vi "Data_get.vi"() -> ()   [LabVIEW 2009]
uses:
  <vilib>/Analysis/2dsp.llb/Real FFT.vi
  <vilib>/Analysis/NI_AALPro.lvlib
panel:
  in  "Substr":bool
  out "tdsavges#":i32 caption="tds averaged:"
  in  "Auto":bool caption="Autosave"
  in  "FFT every#":u32=1 min=1 max=1000 step=1
  in  "#steps":u32=1 min=1 step=1
  in  "f step (MHz)":dbl=0.0003 min=0.00025 max=67.0 step=1e-06 format="%#.12f"
  in  "ps/point":T1(ring)
  in  "ns/div":T2(ring)
  out "Current sweep":u32=1 min=1 max=1000 step=1
  in  "Ext":string="ccd"
  out "f cur. (MHz)":string
  in  "Name":string="trace"
  in  "Folder":path
  in  "#Sweeps":u32=1 min=1 max=1000 step=1
  in  "Ampl. (dBm)":dbl min=-135.0 max=30.0 step=0.5 format="%#_8g"
  in  "f start (MHz)":dbl=0.0003 min=0.00025 max=67.0 step=1e-06 format="%#.12f"
  in  "Start":bool
  in  "Quit":bool
  in  "E8257D VISA Port":refnum<visa-resource-name>="GPIB0::1::INSTR"
  out "read time (ms)":u32
  out "#points":u32
  out "Busy":bool
  in  "Repetition rate (Hz)":ext=2.5
  in  "Chirp start (MHz)":ext=2.5
  in  "Filter up to (MHz)":ext=2.5
  in  "Amount of averagings":u32=10
  out "Data":dbl[](array[numeric])
  out "XY Graph 5":cluster{ext[], dbl[]}(graph)
  out "FFT (Im)":dbl[](array[numeric])
  out "FFT (Re)":dbl[](array[numeric])
  out "Final array":ext[][](array[numeric])
  out "size(s)":i32
  out "Oscilloscope Data":dbl[](array[numeric])
  in  "Channel Number":u16=1
  out "Oscilloscope graph":dbl[](graph)
  in  "Stop":bool
  in  "TDS VISA Port":refnum<visa-resource-name>="GPIB0::1::INSTR"
  # "TDS6000"
  # "E8257D"
  # "File Storage"
  # "Control"
  # "Spectrum data"
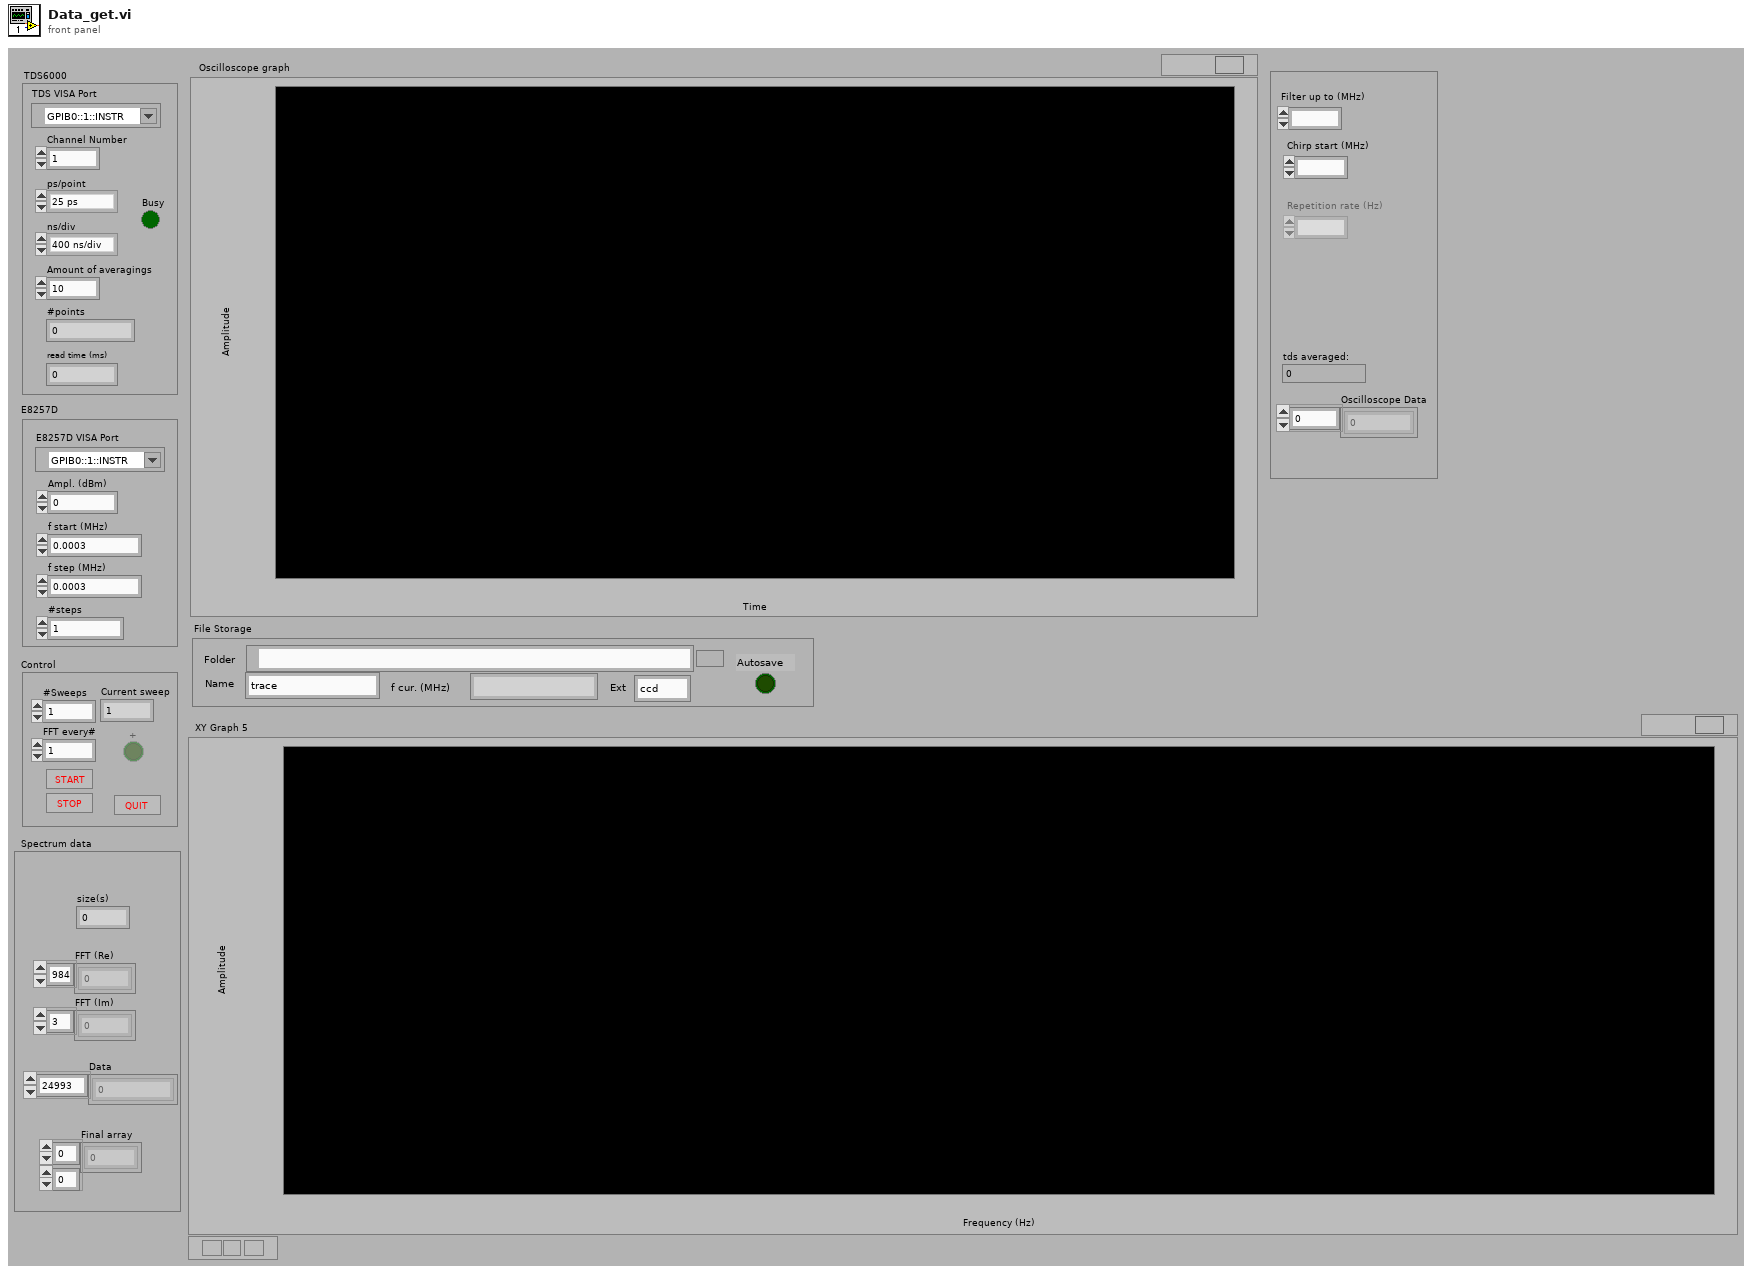
[diagram p1: front panel]
types:
  T1 = enum16{"25 ps", "50 ps", "100 ps", "200 ps", "400 ps", "800 ps", "2 ns"}
  T2 = enum16{"400 ns/div", "1 us/div", "2 us/div", "4 us/div", "10 us/div", "20 us/div"}
  T3 = enum16{"open", "replace", "create", "open or create", "replace or create", "replace or create with confirmation"}
  T4 = cluster{"Folder":path, "Name":string, "Ext":string}
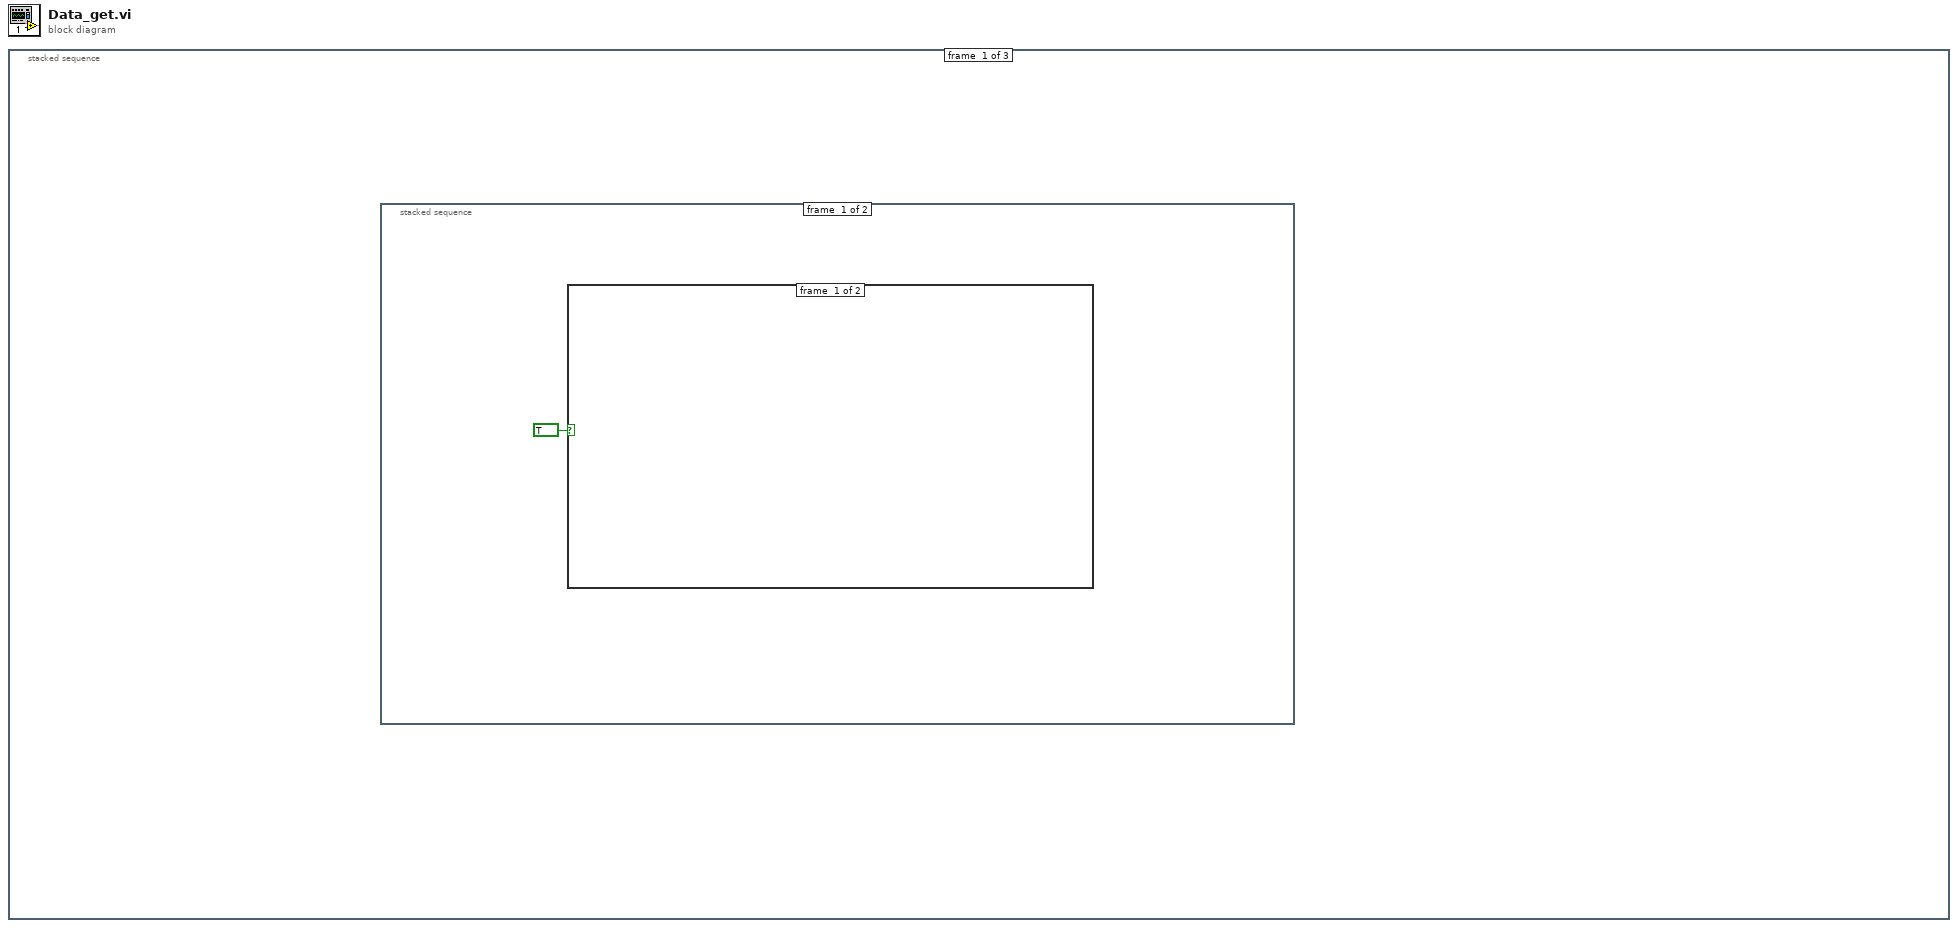
[diagram p0: block diagram]
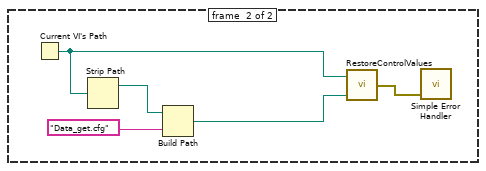
[diagram p2: hidden frame]
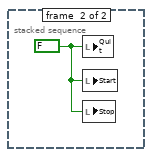
[diagram p3: hidden frame]
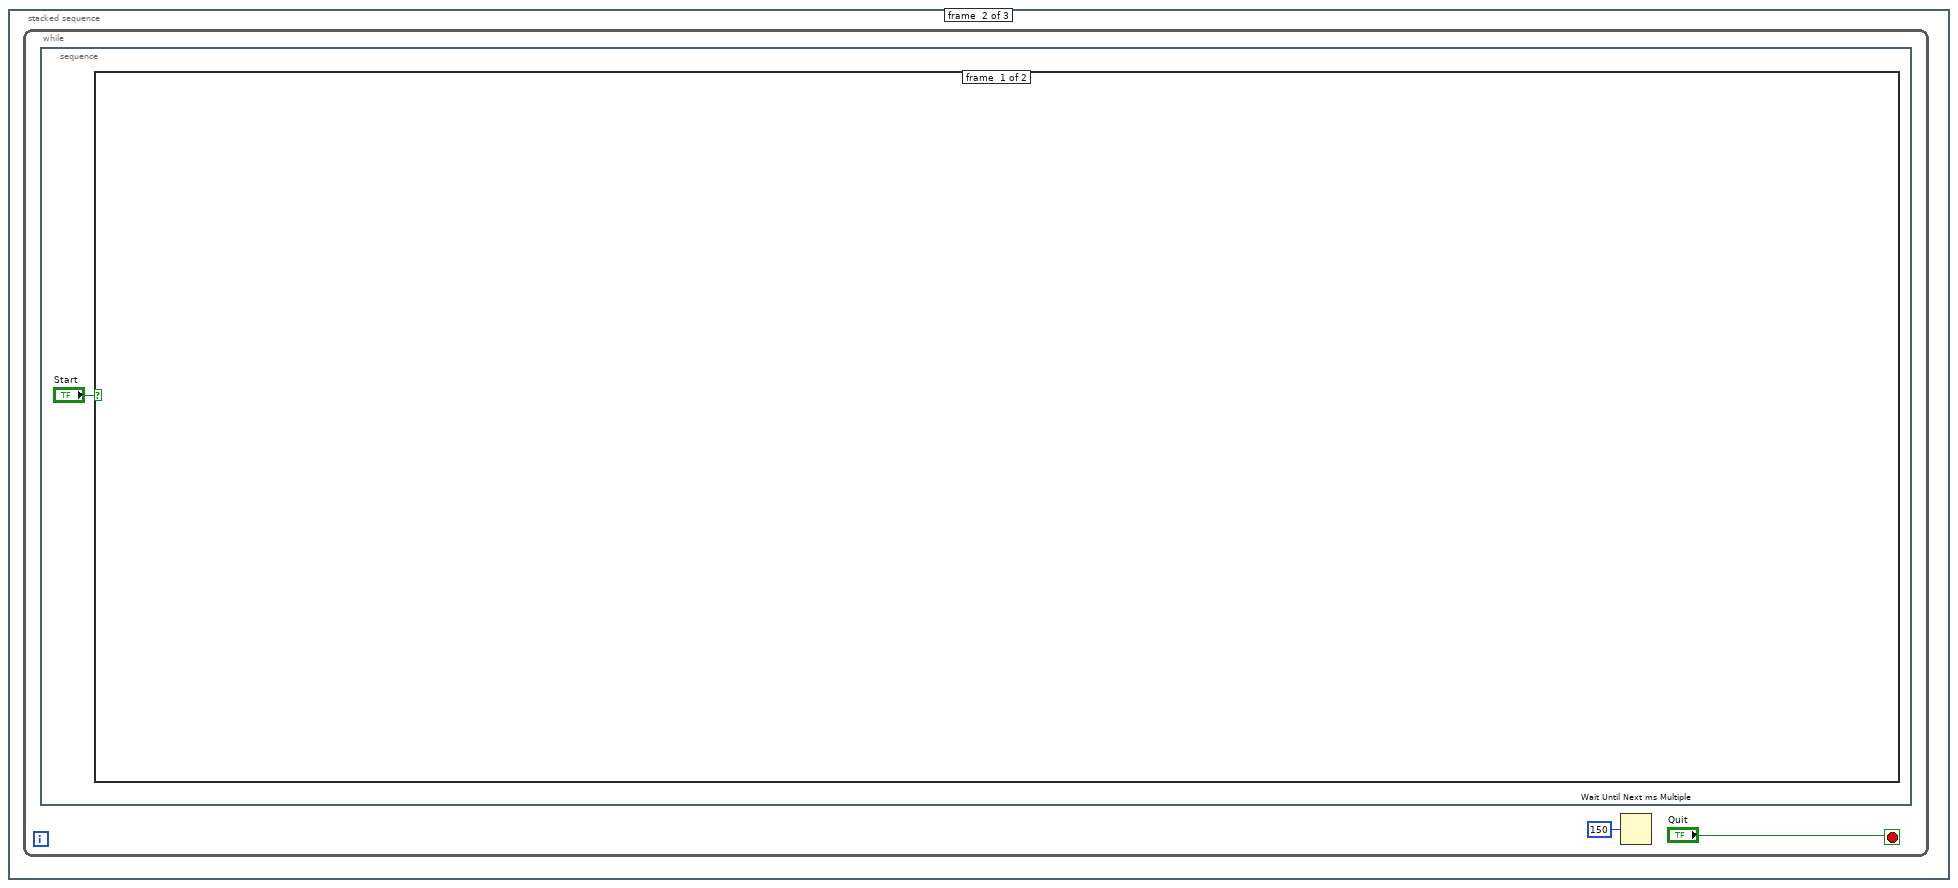
[diagram p4: hidden frame]
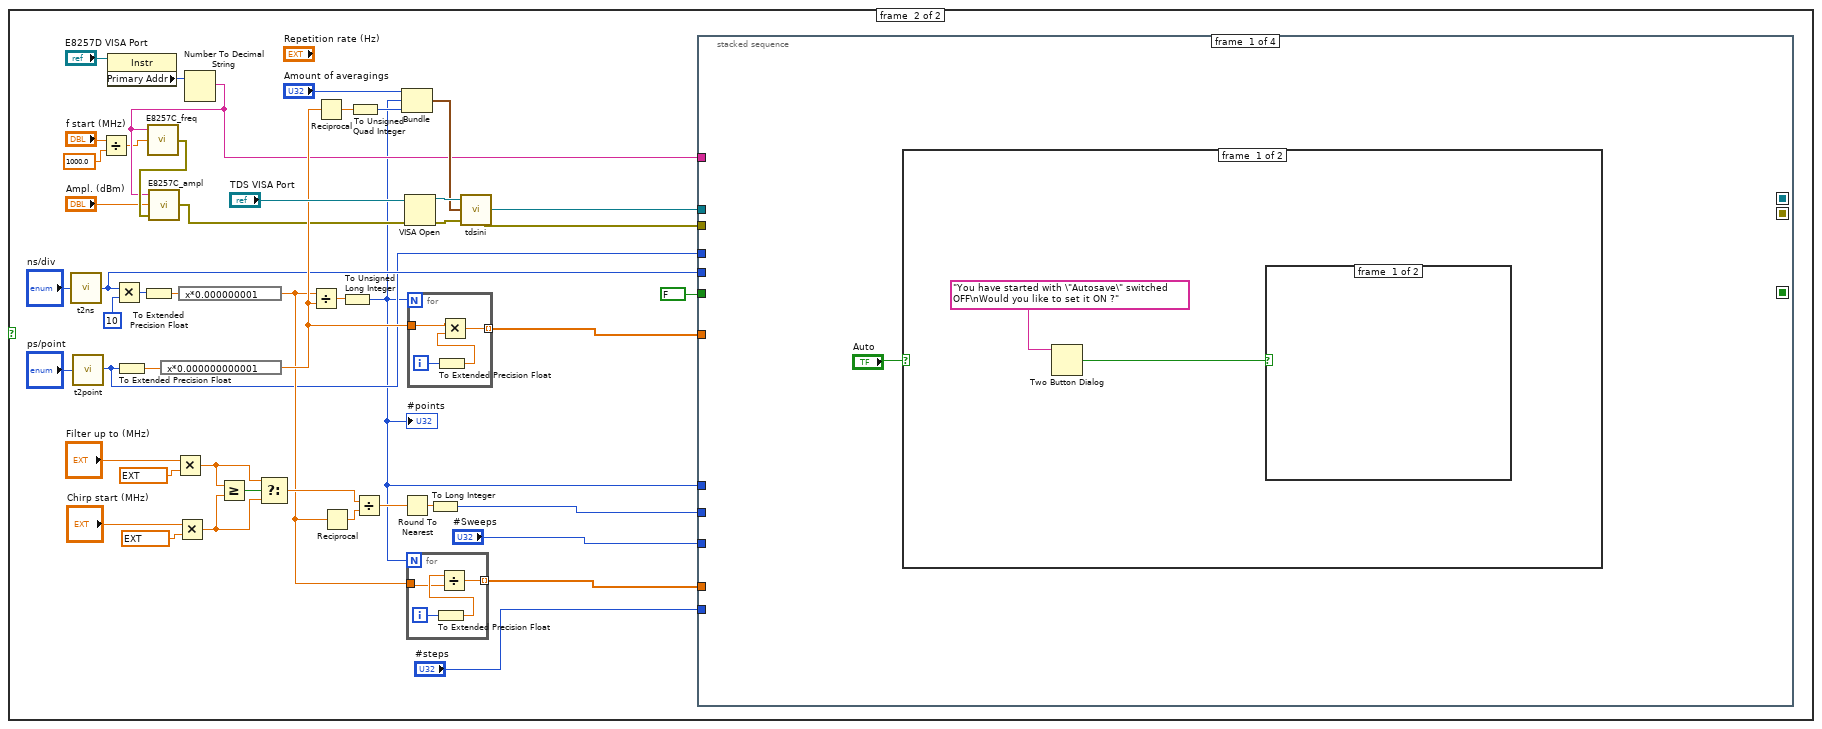
[diagram p5: hidden frame]
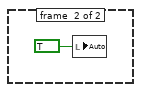
[diagram p6: hidden frame]
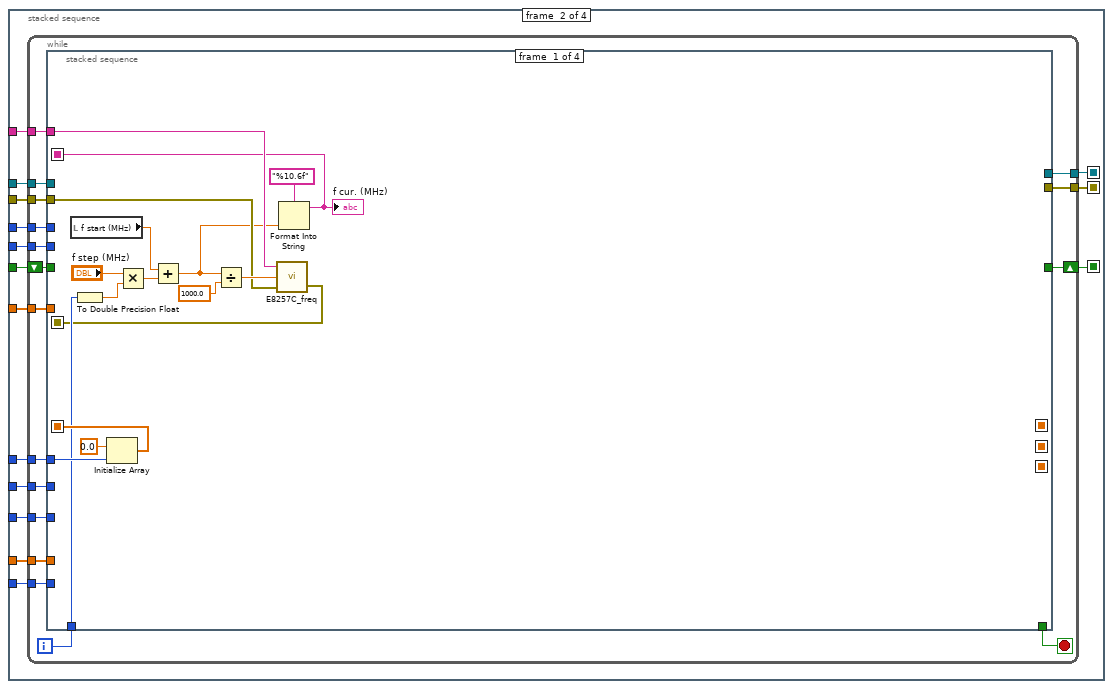
[diagram p8: hidden frame]
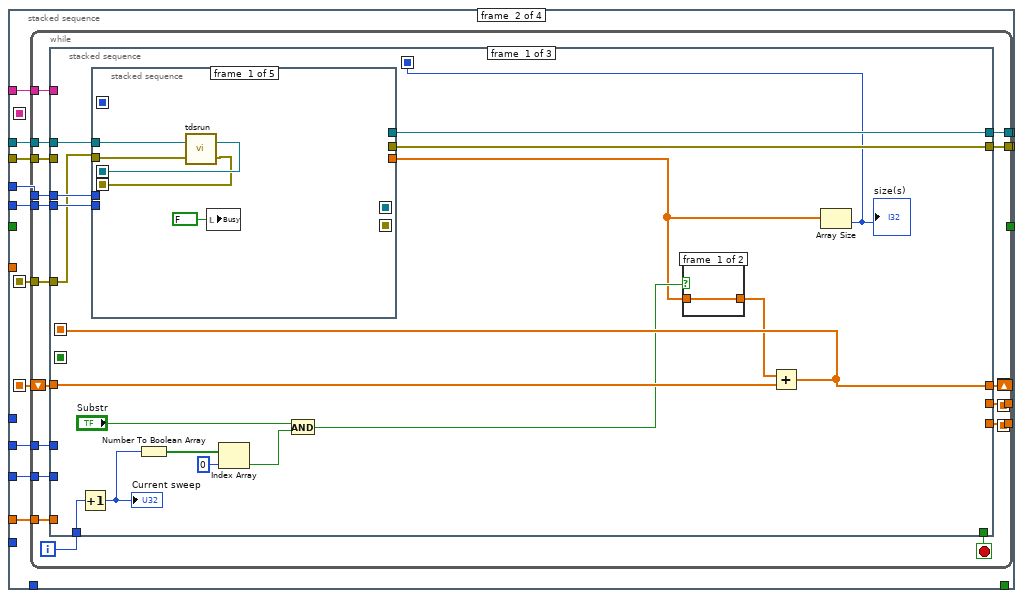
[diagram p9: hidden frame]
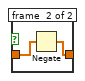
[diagram p10: hidden frame]
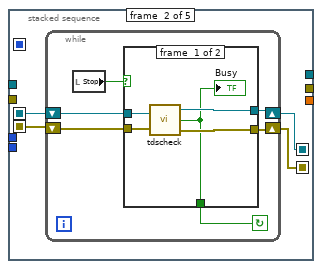
[diagram p11: hidden frame]
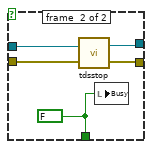
[diagram p12: hidden frame]
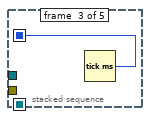
[diagram p13: hidden frame]
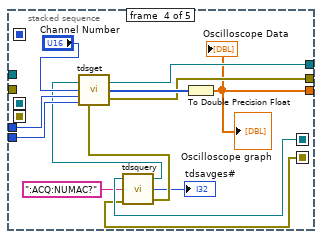
[diagram p14: hidden frame]
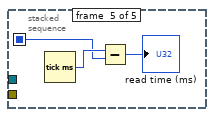
[diagram p15: hidden frame]
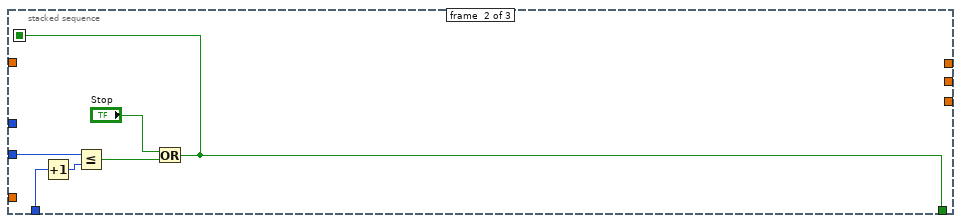
[diagram p16: hidden frame]
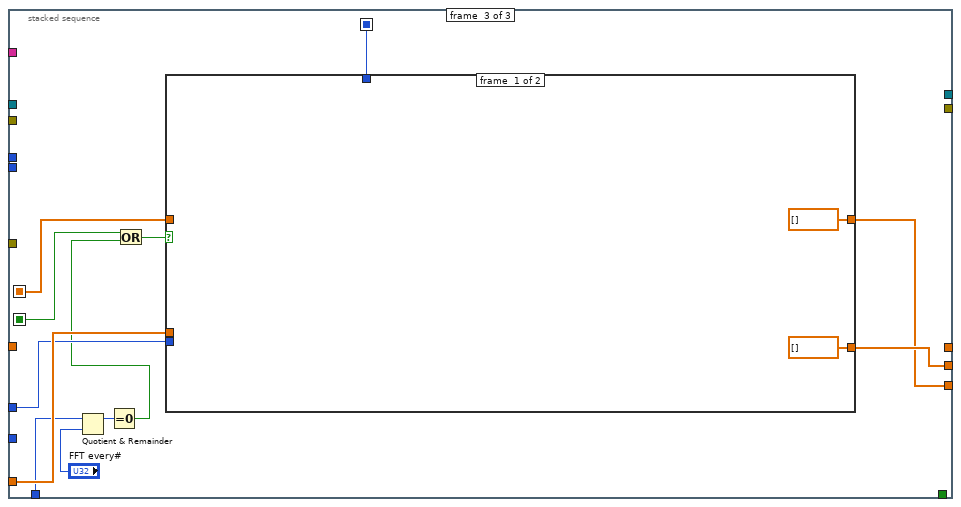
[diagram p17: hidden frame]
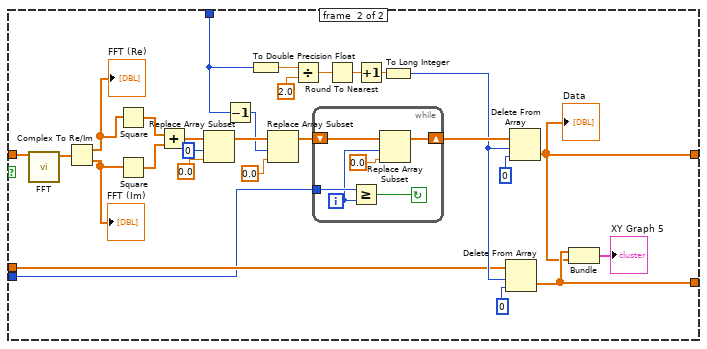
[diagram p18: hidden frame]
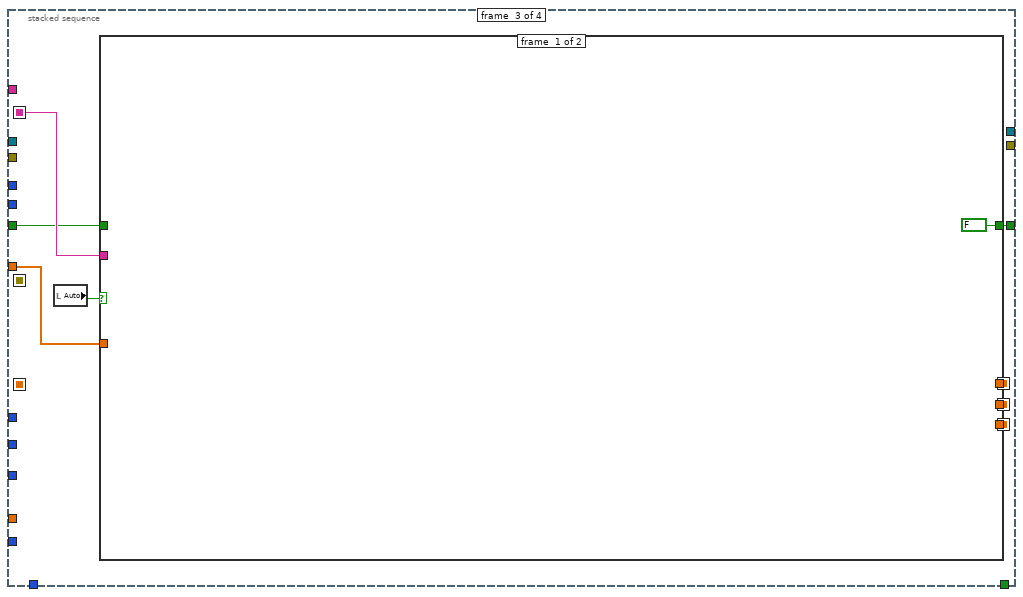
[diagram p19: hidden frame]
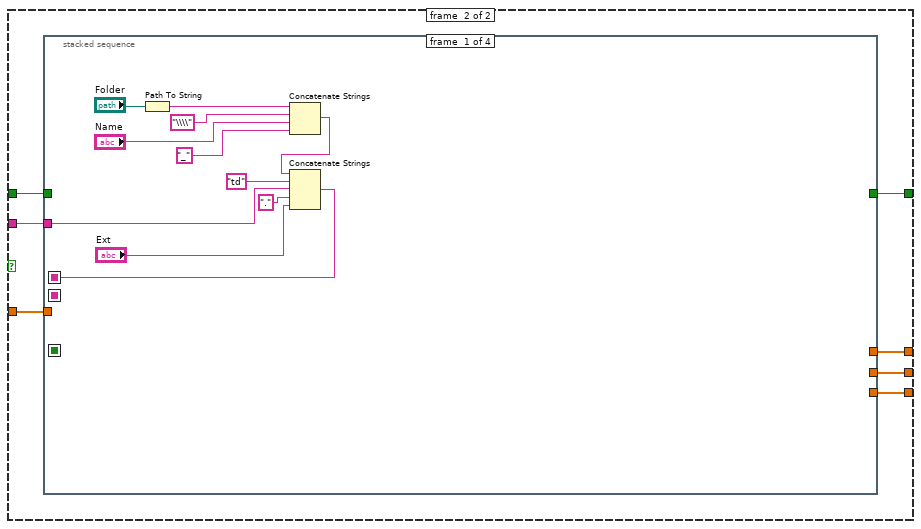
[diagram p20: hidden frame]
diagram:
  n1 = stacked-sequence {
    frame #0 {
      n2 = stacked-sequence {
        frame #0 {
          n3 = case shown="True" TRUE {
            frame #0 {
            }
            frame #1 {
              n4 = Current VI's Path() -> (path=w2:path)
              n5 = Strip Path(path=w2) -> (stripped path=w3:path)  [unwired: 1 out]
              n6 = Build Path(base path=w3, name or relative path="Data_get.cfg") -> (appended path=w5:path)
              n7 = call "RestoreControlValues.vi"("file path"=w5, "vi path"=w2) -> ("error out"=w4:errorcluster)
              n8 = call <vilib>:"Simple Error Handler.vi"("error in (no error)"=w4) -> ()  [unwired: 4 in, 5 out]
            }
          }
        }
        frame #1 {
          w7 = FALSE ("Quit")
          n9 = local write "Quit"(w7) -> ()
          n10 = local write "Start"(w7) -> ()
          n11 = local write "Stop"(w7) -> ()
        }
      }
    }
    frame #1 {
      n12 = while {
        stop <- "Quit" stop-if-true
        n13 = stacked-sequence {
          frame #0 {
            n14 = case shown="True" "Start" {
              frame #0 {
              }
              frame #1 {
                n15 = call "t2ns.vi"("t/div"="ns/div") -> ("ns/div"=w17:u32)
                n16 = call "t2point.vi"("t/point"="ps/point") -> ("ps/point"=w15:u32)
                n17 = Divide(x="f start (MHz)", y=1000.0) -> (x/y=w20:dbl)
                n18 = property class="Instr"(reference="E8257D VISA Port") -> ("Primary Addr"=w27:u16)  [unwired: 1 in, 2 out]
                n19 = Multiply(x=w17, y=u32 10) -> (x*y=w51:u32)
                n20 = To Extended Precision Float(1:w15) -> (0:w48:ext)
                n21 = To Extended Precision Float(1:w51) -> (0:w49:ext)
                n22 = expression code="x*0.000000000001"(w48) -> (w33:ext)
                n23 = Multiply(x="Filter up to (MHz)", y=ext 1000000.0) -> (x*y=w39:ext)
                n24 = Multiply(x="Chirp start (MHz)", y=ext 1000000.0) -> (x*y=w36:ext)
                n25 = expression code="x*0.000000001"(w49) -> (w29:ext)
                n26 = Number To Decimal String(number=w27) -> (decimal integer string=w24:string)  [unwired: 1 in]
                n27 = call "E8257C_freq.vi"("Frequency GHz"=w20, "GPIB address"=w24) -> ("error out"=w25:errorcluster)  [unwired: 1 in]
                n28 = call "E8257C_ampl.vi"("error in"=w25, "Amplitude dBm"="Ampl. (dBm)", "GPIB address"=w24) -> ("error out"=w23:errorcluster)
                n29 = Greater Or Equal?(x=w39, y=w36) -> (x >= y?=w47:bool)
                n30 = Select(t=w39, s=w47, f=w36) -> (s? t:f=w45:ext)
                n31 = Divide(x=w29, y=w33) -> (x/y=w50:ext)
                n32 = Reciprocal(x=w33) -> (1/x=w31:ext)
                n33 = Reciprocal(x=w29) -> (1/x=w46:ext)
                n34 = To Unsigned Long Integer(number=w50) -> (unsigned 32bit integer=w13:u32)
                "#points" <- w13
                n35 = To Unsigned Quad Integer(1:w31) -> (0:w32:u64)
                n36 = Divide(x=w45, y=w46) -> (x/y=w44:ext)
                n37 = Bundle("Amount of averagings"="Amount of averagings", w13, w32) -> (w34:cluster{"Amount of averagings ":u32, u32, u64})  [unwired: 1 in]
                n38 = Round To Nearest(number=w44) -> (nearest integer value=w43:ext)
                n39 = VISA Open(error in (no error)=w23, VISA resource name="TDS VISA Port") -> (VISA resource name=w54:refnum<visa-resource-name>, error out=w55:errorcluster)  [unwired: 3 in]
                n40 = for {
                  N: w13 -> [_]
                  tunnel: w29 -> [w433]
                  tunnel: [w435] -> w30 mode=indexing
                  i -> [w436]
                  n41 = To Extended Precision Float(1:w436) -> (0:w434:ext)
                  n42 = Divide(x=w434, y=w433) -> (x/y=w435:ext)
                }
                n43 = for {
                  N: w13 -> [_]
                  tunnel: w33 -> [w438]
                  tunnel: [w437] -> w18 mode=indexing
                  i -> [w440]
                  n44 = To Extended Precision Float(1:w440) -> (0:w439:ext)
                  n45 = Multiply(x=w438, y=w439) -> (x*y=w437:ext)
                }
                n46 = To Long Integer(number=w43) -> (32bit integer=w42:i32)
                n47 = call "tdsini.vi"("Error In (No Error)"=w55, "Acq_par"=w34, "VISA Port In"=w54) -> ("Error Out"=w56:errorcluster, "VISA Port Out"=w57:refnum<visa-resource-name>)
                n48 = stacked-sequence {
                  seq-local: [_ w68 _ _] -> [_ _ w394 _]
                  seq-local: [_ w67 _ _] -> [_ _ w393 _]
                  seq-local: [_ w62 _ _] -> [_ _ _ w395]
                  tunnel: w57 -> [_ w76 _ _]
                  tunnel: w56 -> [_ w75 _ _]
                  tunnel: w15 -> [_ w74 _ _]
                  tunnel: w17 -> [_ w73 _ _]
                  tunnel: w42 -> [_ w72 _ _]
                  tunnel: w30 -> [_ w71 _ _]
                  tunnel: w24 -> [_ w70 w391 _]
                  tunnel: "#Sweeps" -> [_ w69 _ _]
                  tunnel: w18 -> [_ w64 _ _]
                  tunnel: w13 -> [_ w66 _ _]
                  tunnel: "#steps" -> [_ w65 _ _]
                  tunnel: FALSE -> [_ w63 _ _]
                  frame #0 {
                    n49 = case shown="False" "Auto" {
                      frame #0 {
                        n50 = Two Button Dialog(message="You have started with \"Autosave\" switched OFF\nWould you like to set it ON ?") -> (T button?=w59:bool)  [unwired: 2 in]
                        n51 = case shown="True" w59 {
                          frame #0 {
                          }
                          frame #1 {
                            n52 = local write "Auto"(TRUE) -> ()
                          }
                        }
                      }
                      frame #1 {
                      }
                    }
                  }
                  frame #1 {
                    n53 = while {
                      tunnel: w76 -> [w93]
                      tunnel: w75 -> [w92]
                      tunnel: w74 -> [w91]
                      tunnel: w73 -> [w90]
                      tunnel: w72 -> [w89]
                      tunnel: w71 -> [w88]
                      tunnel: w70 -> [w87]
                      tunnel: w69 -> [w86]
                      tunnel: [w85] -> w68
                      tunnel: [w84] -> w67
                      tunnel: w66 -> [w83]
                      tunnel: w65 -> [w81]
                      tunnel: w64 -> [w79]
                      shift-right: [w77] -> w62
                      shift-left: w63 -> [w78]
                      i -> [w82]
                      stop <- w80 stop-if-true
                      n54 = stacked-sequence {
                        seq-local: [w108 _ _ _] -> [_ w114 _ _]
                        seq-local: [w97 _ _ _] -> [_ w113 _ _]
                        seq-local: [_ w112 _ _] -> [_ _ w265 _]
                        seq-local: [_ w111 _ _] -> [_ _ w264 _]
                        seq-local: [_ w110 _ _] -> [_ _ w263 _]
                        seq-local: [w94 _ _ _] -> [_ _ w262 _]
                        tunnel: w93 -> [_ w124 _ _]
                        tunnel: w92 -> [w98 w123 _ _]
                        tunnel: w91 -> [_ w122 _ _]
                        tunnel: w90 -> [_ w121 _ _]
                        tunnel: w89 -> [_ w120 _ _]
                        tunnel: w88 -> [_ w119 _ _]
                        tunnel: w87 -> [w99 w118 _ _]
                        tunnel: w86 -> [_ w117 _ _]
                        tunnel: [_ w116 _ _] -> w85
                        tunnel: [_ w115 _ _] -> w84
                        tunnel: w83 -> [w107 _ _ _]
                        tunnel: w82 -> [w102 _ _ w387]
                        tunnel: w81 -> [_ _ _ w386]
                        tunnel: [_ _ _ w385] -> w80
                        tunnel: w79 -> [_ _ w266 _]
                        tunnel: w78 -> [_ _ w260 _]
                        tunnel: [_ _ w259 _] -> w77
                        frame #0 {
                          n55 = local read "f start (MHz)"() -> (w100:dbl)
                          n56 = To Double Precision Float(number=w102) -> (double precision float=w103:dbl)
                          n57 = Initialize Array(0.0 ("element"), w107) -> (w108:dbl[])
                          n58 = Multiply(x="f step (MHz)", y=w103) -> (x*y=w101:dbl)
                          n59 = Add(x=w100, y=w101) -> (x+y=w96:dbl)
                          n60 = Divide(x=w96, y=1000.0) -> (x/y=w106:dbl)
                          n61 = call "E8257C_freq.vi"("error in"=w98, "Frequency GHz"=w106, "GPIB address"=w99) -> ("error out"=w97:errorcluster)
                          n62 = Format Into String(format string="%10.6f", w96) -> (resulting string=w94:string)  [unwired: 2 in, 1 out]
                          "f cur. (MHz)" <- w94
                        }
                        frame #1 {
                          n63 = while {
                            tunnel: [w138] -> w115
                            tunnel: [w139] -> w116
                            tunnel: w123 -> [w140]
                            tunnel: w124 -> [w141]
                            tunnel: w122 -> [w137]
                            tunnel: w121 -> [w136]
                            tunnel: w119 -> [w134]
                            tunnel: w120 -> [w135]
                            tunnel: w118 -> [w131]
                            tunnel: w117 -> [w130]
                            shift-right: [w128] -> w112
                            shift-left: w114 -> [w129]
                            tunnel: [w127] -> w111
                            tunnel: w113 -> [w126]
                            tunnel: [w125] -> w110
                            i -> [w133]
                            stop <- w132 stop-if-true
                            n64 = stacked-sequence {
                              seq-local: [w151 _ _] -> [_ _ w222]
                              seq-local: [w152 _ _] -> [_ _ w221]
                              seq-local: [_ w205 _] -> [_ _ w212]
                              tunnel: w141 -> [w159 _ _]
                              tunnel: w140 -> [_ _ _]
                              tunnel: [w158 _ _] -> w139
                              tunnel: [w157 _ _] -> w138
                              tunnel: w137 -> [w156 _ _]
                              tunnel: w136 -> [w155 _ _]
                              tunnel: w135 -> [_ _ w219]
                              tunnel: w134 -> [_ _ w220]
                              tunnel: w133 -> [w150 w210 w216]
                              tunnel: [_ w205 _] -> w132
                              tunnel: w131 -> [_ _ _]
                              tunnel: w130 -> [_ w207 _]
                              tunnel: w129 -> [w154 _ _]
                              tunnel: [w152 _ _] -> w128
                              tunnel: [_ _ w218] -> w127
                              tunnel: w126 -> [w153 _ _]
                              tunnel: [_ _ w217] -> w125
                              frame #0 {
                                n65 = Increment(x=w150) -> (x+1=w142:i32)
                                "Current sweep" <- w142
                                n66 = stacked-sequence {
                                seq-local: [w165 _ _ _ _] -> [_ w171 _ _ _]
                                seq-local: [w164 _ _ _ _] -> [_ w170 _ _ _]
                                seq-local: [_ w168 _ _ _] -> [_ _ _ w193 _]
                                seq-local: [_ w169 _ _ _] -> [_ _ _ w194 _]
                                seq-local: [_ _ w188 _ _] -> [_ _ _ _ w203]
                                tunnel: w159 -> [w166 _ _ _ _]
                                tunnel: w153 -> [w167 _ _ _ _]
                                tunnel: [_ _ _ w200 _] -> w158
                                tunnel: [_ _ _ w199 _] -> w157
                                tunnel: w156 -> [_ _ _ w197 _]
                                tunnel: w155 -> [_ _ _ w196 _]
                                tunnel: [_ _ _ w195 _] -> w145
                                frame #0 {
                                n67 = call "tdsrun.vi"("Error In (No Error)"=w167, "VISA Port In"=w166) -> ("Error Out"=w164:errorcluster, "VISA Port Out"=w165:refnum<visa-resource-name>)
                                n68 = local write "Busy"(FALSE ("Busy")) -> ()
                                }
                                frame #1 {
                                n69 = while {
                                shift-right: [w175] -> w169
                                shift-left: w171 -> [w176]
                                shift-right: [w174] -> w168
                                shift-left: w170 -> [w177]
                                stop <- w173 continue-if-true
                                n70 = local read "Stop"() -> (w172:bool)
                                n71 = case shown="True" w172 {
                                tunnel: w177 -> [w182 w186]
                                tunnel: w176 -> [w181 w187]
                                tunnel: [w180 w184] -> w175
                                tunnel: [w179 w185] -> w174
                                tunnel: [w178 w183] -> w173
                                frame #0 {
                                n72 = call "tdscheck.vi"("VISA Port In"=w181, "Error In (No Error)"=w182) -> ("VISA Port Out"=w180:refnum<visa-resource-name>, "busy"=w178:bool, "Error Out"=w179:errorcluster)
                                "Busy" <- w178
                                }
                                frame #1 {
                                w183 = FALSE ("busy")
                                n73 = call "tdsstop.vi"("Error In (No Error)"=w186, "VISA Port In"=w187) -> ("Error Out"=w185:errorcluster, "VISA Port Out"=w184:refnum<visa-resource-name>)
                                n74 = local write "Busy"(w183) -> ()
                                }
                                }
                                }
                                }
                                frame #2 {
                                n75 = Tick Count (ms)() -> (millisecond timer value=w188:u32)
                                }
                                frame #3 {
                                n76 = call "tdsquery.vi"("Error In (No Error)"=w193, "String to TDS"=":ACQ:NUMAC?", "VISA Port In"=w194) -> ("Error Out"=w190:errorcluster, "number"=→"tdsavges#":i32, "VISA Port Out"=w191:refnum<visa-resource-name>)
                                n77 = call "tdsget.vi"("VISA Port In"=w191, "Channel Number"="Channel Number", "ps/point"=w197, "ns/div"=w196, "Error In (No Error)"=w190) -> ("VISA Port Out"=w200:refnum<visa-resource-name>, "TDS Data"=w201:u16[], "Error Out"=w199:errorcluster)  [unwired: 8 in]
                                n78 = To Double Precision Float(number=w201) -> (double precision float=w195:dbl[])
                                "Oscilloscope graph" <- w195
                                "Oscilloscope Data" <- w195
                                }
                                frame #4 {
                                n79 = Tick Count (ms)() -> (millisecond timer value=w204:u32)
                                n80 = Subtract(x=w204, y=w203) -> (x-y=→"read time (ms)":u32)
                                }
                                }
                                n81 = Number To Boolean Array(number=w142) -> (Boolean array=w149:bool[])
                                n82 = Index Array(array=w149, index=0) -> (element=w147:bool)
                                n83 = And(x="Substr", y=w147) -> (x .and. y?=w146:bool)
                                n84 = case shown="True" w146 {
                                tunnel: w145 -> [w160 w162]
                                tunnel: [w160 w161] -> w144
                                frame #0 {
                                }
                                frame #1 {
                                n85 = Negate(x=w162) -> (-x=w161:dbl[])
                                }
                                }
                                n86 = Add(x=w144, y=w154) -> (x+y=w152:dbl[])
                                n87 = Array Size(array=w145) -> (size(s)=w151:i32)
                                "size(s)" <- w151
                              }
                              frame #1 {
                                n88 = Increment(x=w210) -> (x+1=w206:i32)
                                n89 = Less Or Equal?(x=w207, y=w206) -> (x <= y?=w209:bool)
                                n90 = Or(x="Stop", y=w209) -> (x .or. y?=w205:bool)
                              }
                              frame #2 {
                                n91 = Quotient & Remainder(x=w216, y="FFT every#") -> (x-y*floor(x/y)=w214:u32)  [unwired: 1 out]
                                n92 = Equal To 0?(x=w214) -> (x = 0?=w211:bool)
                                n93 = Or(x=w212, y=w211) -> (x .or. y?=w213:bool)
                                n94 = case shown="True" w213 {
                                tunnel: w222 -> [_ w230]
                                tunnel: w221 -> [_ w229]
                                tunnel: w220 -> [_ w228]
                                tunnel: w219 -> [_ w227]
                                tunnel: [ext[] [] w226] -> w218
                                tunnel: [dbl[] [] w225] -> w217
                                frame #0 {
                                }
                                frame #1 {
                                n95 = call-poly <vilib>:"FFT.vi"("X"=w229) -> ("FFT {X}"=w252:cdb[])  [unwired: 9 in, 1 out]
                                n96 = Complex To Re/Im(x + iy=w252) -> (x=w251:dbl[], y=w250:dbl[])
                                "FFT (Re)" <- w251
                                "FFT (Im)" <- w250
                                n97 = Square(x=w251) -> (x^2=w249:dbl[])
                                n98 = Square(x=w250) -> (x^2=w248:dbl[])
                                n99 = Add(x=w249, y=w248) -> (x+y=w244:dbl[])
                                n100 = Replace Array Subset(array=w244, new element=0.0 ("new element/subarray"), index=0) -> (w243:dbl[])
                                n101 = Decrement(x=w230) -> (x-1=w242:i32)
                                n102 = To Double Precision Float(number=w230) -> (double precision float=w238:dbl)
                                n103 = Replace Array Subset(array=w243, new element=0.0 ("new element/subarray"), index=w242) -> (w240:dbl[])
                                n104 = Divide(x=w238, y=2.0) -> (x/y=w236:dbl)
                                n105 = while {
                                tunnel: w227 -> [w257]
                                shift-right: [w255] -> w239
                                shift-left: w240 -> [w256]
                                i -> [w254]
                                stop <- w258 continue-if-true
                                n106 = Greater Or Equal?(x=w257, y=w254) -> (x >= y?=w258:bool)
                                n107 = Replace Array Subset(array=w256, new element=0.0 ("new element/subarray"), index=w254) -> (w255:dbl[])
                                }
                                n108 = Round To Nearest(number=w236) -> (nearest integer value=w235:dbl)
                                n109 = Increment(x=w235) -> (x+1=w234:dbl)
                                n110 = To Long Integer(number=w234) -> (32bit integer=w231:i32)
                                n111 = Delete From Array(array=w228, length=w231, index=0) -> (deleted portion=w226:ext[])  [unwired: 1 out]
                                n112 = Delete From Array(array=w239, length=w231, index=0) -> (deleted portion=w225:dbl[])  [unwired: 1 out]
                                "Data" <- w225
                                n113 = Bundle(w226, w225) -> (→"XY Graph 5":cluster{ext[], dbl[]})  [unwired: 1 in]
                                }
                                }
                              }
                            }
                          }
                        }
                        frame #2 {
                          n114 = local read "Auto"() -> (w261:bool)
                          n115 = case shown="True" w261 {
                            tunnel: w266 -> [_ w274]
                            tunnel: w265 -> [_ w273]
                            tunnel: w264 -> [_ w272]
                            tunnel: w263 -> [_ w271]
                            tunnel: w262 -> [_ w270]
                            tunnel: w260 -> [_ w269]
                            tunnel: [FALSE w268] -> w259
                            frame #0 {
                            }
                            frame #1 {
                              n116 = stacked-sequence {
                                seq-local: [w275 _ _ _] -> [_ w300 _ _]
                                seq-local: [_ _ w355 _] -> [_ _ _ w376]
                                seq-local: [_ w287 _ _] -> [_ _ _ w367]
                                tunnel: w274 -> [_ w302 _ _]
                                tunnel: w273 -> [_ w289 _ _]
                                tunnel: w272 -> [_ _ _ w379]
                                tunnel: w271 -> [_ _ _ w378]
                                tunnel: w270 -> [w277 w288 w357 _]
                                tunnel: w269 -> [_ w292 _ _]
                                tunnel: [_ w287 _ _] -> w268
                                frame #0 {
                                n117 = Path To String(path="Folder") -> (string=w285:string)
                                n118 = Concatenate Strings(w285, "\\\\" ("string"), "Name", "_") -> (w276:string)
                                n119 = Concatenate Strings(w276, "td", w277, ".", "Ext") -> (w275:string)
                                }
                                frame #1 {
                                n120 = String To Path(string=w300) -> (path=w291:path)
                                n121 = case shown="False" w292 {
                                tunnel: w300 -> [w306 _]
                                tunnel: [w311 w353] -> w287
                                tunnel: [w309 T3."replace or create" ("operation (0:open)")] -> w294
                                tunnel: w292 -> [w310 w353]
                                tunnel: w291 -> [w308 w352]
                                tunnel: [w307 w352] -> w290
                                tunnel: w288 -> [w305 _]
                                frame #0 {
                                n122 = call "CheckFileExist.vi"("Path"=w306) -> ("Exist"=w313:bool, "Overwrite"=w312:bool)  [unwired: 1 in, 1 out]
                                n123 = case shown="True" w313 {
                                tunnel: w312 -> [_ w322]
                                tunnel: [w316 w320] -> w311
                                tunnel: w310 -> [w316 _]
                                tunnel: [T3."create" ("operation (0:open)") w321] -> w309
                                tunnel: w308 -> [w314 w319]
                                tunnel: [w314 w318] -> w307
                                tunnel: w305 -> [_ w317]
                                frame #0 {
                                }
                                frame #1 {
                                n124 = case shown="True" w322 {
                                tunnel: [w325 T3."replace or create" ("operation (0:open)")] -> w321
                                tunnel: [w326 TRUE] -> w320
                                tunnel: w319 -> [_ w349]
                                tunnel: [w323 w349] -> w318
                                tunnel: w317 -> [w324 _]
                                frame #0 {
                                n125 = stacked-sequence {
                                tunnel: [_ _ FALSE] -> w326
                                tunnel: [_ _ T3."create" ("operation (0:open)")] -> w325
                                tunnel: w324 -> [_ w338 _]
                                tunnel: [_ w335 _] -> w323
                                frame #0 {
                                n126 = local read "Folder"() -> (w334:path)
                                n127 = local read "Name"() -> (w333:string)
                                n128 = local read "Ext"() -> (w332:string)
                                n129 = Bundle("Folder"=w334, "Name"=w333, "Ext"=w332) -> (w331:T4)  [unwired: 1 in]
                                n130 = call "ChangeFileName.vi"("input par"=w331) -> ("output par"=w330:T4)  [unwired: 1 out]
                                n131 = Unbundle(w330) -> ("Folder"=w329:path, "Name"=w328:string, "Ext"=w327:string)
                                n132 = local write "Folder"(w329) -> ()
                                n133 = local write "Name"(w328) -> ()
                                n134 = local write "Ext"(w327) -> ()
                                }
                                frame #1 {
                                n135 = local read "Folder"() -> (w343:path)
                                n136 = local read "Name"() -> (w342:string)
                                n137 = local read "Ext"() -> (w337:string)
                                n138 = Path To String(path=w343) -> (string=w346:string)
                                n139 = Concatenate Strings(w346, "\\\\" ("string"), w342, "_") -> (w339:string)
                                n140 = Concatenate Strings(w339, "td", w338, ".", w337) -> (w336:string)
                                n141 = String To Path(string=w336) -> (path=w335:path)
                                }
                                frame #2 {
                                }
                                }
                                }
                                frame #1 {
                                }
                                }
                                }
                                }
                                }
                                frame #1 {
                                }
                                }
                                n142 = Build Array(w302, w289) -> (w304:ext[][])
                                n143 = Transpose 2D Array(2D array=w304) -> (transposed array=w301:ext[][])
                                n144 = Array To Spreadsheet String(array=w301, 3:"%e") -> (spreadsheet string=w293:string)  [unwired: 1 in]
                                n145 = Open/Create/Replace File(file path (use dialog)=w290, operation (0:open)=w294, access (0:read/write)=enum16{"read/write", "read-only", "write-only"}."write-only") -> (refnum out=w296:refnum<file>, error out=w299:errorcluster)  [unwired: 3 in, 1 out]
                                n146 = Write to Text File(file (use dialog)=w296, text=w293, error in=w299) -> (refnum out=w297:refnum<file>, error out=w298:errorcluster)  [unwired: 1 in, 1 out]
                                n147 = Close File(refnum=w297, error in=w298) -> (error out=w286:errorcluster)  [unwired: 1 out]
                                n148 = call <vilib>:"Simple Error Handler.vi"("error in (no error)"=w286) -> ()  [unwired: 4 in, 5 out]
                                }
                                frame #2 {
                                n149 = local read "Folder"() -> (w359:path)
                                n150 = local read "Name"() -> (w358:string)
                                n151 = local read "Ext"() -> (w356:string)
                                n152 = Path To String(path=w359) -> (string=w365:string)
                                n153 = Concatenate Strings(w365, "\\\\" ("string"), w358, "_") -> (w360:string)
                                n154 = Concatenate Strings(w360, "sd", w357, ".", w356) -> (w355:string)
                                }
                                frame #3 {
                                n155 = To Extended Precision Float(1:w378) -> (0:w380:ext[])
                                n156 = String To Path(string=w376) -> (path=w369:path)
                                n157 = case shown="True" w367 {
                                tunnel: [T3."replace or create with confirmation" ("operation (0:open)") T3."replace or create" ("operation (0:open)")] -> w368
                                frame #0 {
                                }
                                frame #1 {
                                }
                                }
                                n158 = Build Array(w379, w380) -> (w377:ext[][])
                                n159 = Transpose 2D Array(2D array=w377) -> (transposed array=w381:ext[][])
                                "Final array" <- w381
                                n160 = Array To Spreadsheet String(array=w381, 3:"%e") -> (spreadsheet string=w370:string)  [unwired: 1 in]
                                n161 = Open/Create/Replace File(file path (use dialog)=w369, operation (0:open)=w368, access (0:read/write)=enum16{"read/write", "read-only", "write-only"}."write-only") -> (refnum out=w372:refnum<file>, error out=w375:errorcluster)  [unwired: 3 in, 1 out]
                                n162 = Write to Text File(file (use dialog)=w372, text=w370, error in=w375) -> (refnum out=w373:refnum<file>, error out=w374:errorcluster)  [unwired: 1 in, 1 out]
                                n163 = Close File(refnum=w373, error in=w374) -> (error out=w366:errorcluster)  [unwired: 1 out]
                                n164 = call <vilib>:"Simple Error Handler.vi"("error in (no error)"=w366) -> ()  [unwired: 4 in, 5 out]
                                }
                              }
                            }
                          }
                        }
                        frame #3 {
                          n165 = Increment(x=w387) -> (x+1=w389:i32)
                          n166 = Less Or Equal?(x=w386, y=w389) -> (x <= y?=w390:bool)
                          n167 = local read "Stop"() -> (w388:bool)
                          n168 = Or(x=w388, y=w390) -> (x .or. y?=w385:bool)
                        }
                      }
                    }
                  }
                  frame #2 {
                    n169 = call "E8257C_local.vi"("GPIB address"=w391) -> ("error out"=w392:errorcluster)  [unwired: 1 in]
                    n170 = call <vilib>:"Simple Error Handler.vi"("error in (no error)"=w392) -> ()  [unwired: 4 in, 5 out]
                    n171 = VISA Close(VISA resource name=w394, error in (no error)=w393) -> ()  [unwired: 1 out]
                  }
                  frame #3 {
                    n172 = local read "Auto"() -> (w396:bool)
                    n173 = case shown="True" w396 {
                      tunnel: w395 -> [_ w399]
                      frame #0 {
                      }
                      frame #1 {
                        n174 = local read "Channel Number"() -> (w429:u16)
                        n175 = local read "ps/point"() -> (w428:T1)
                        n176 = local read "ns/div"() -> (w427:T2)
                        n177 = local read "Amount of averagings"() -> (w426:u32)
                        n178 = local read "#Sweeps"() -> (w425:u32)
                        n179 = local read "Filter up to (MHz)"() -> (w424:ext)
                        n180 = local read "Chirp start (MHz)"() -> (w423:ext)
                        n181 = local read "Ampl. (dBm)"() -> (w422:dbl)
                        n182 = local read "f start (MHz)"() -> (w419:dbl)
                        n183 = local read "f step (MHz)"() -> (w418:dbl)
                        n184 = local read "#steps"() -> (w417:u32)
                        n185 = call "t2point.vi"("t/point"=w428) -> ("ps/point"=w420:u32)
                        n186 = call "t2ns.vi"("t/div"=w427) -> ("ns/div"=w421:u32)
                        n187 = local read "Folder"() -> (w413:path)
                        n188 = local read "Name"() -> (w412:string)
                        n189 = local read "Ext"() -> (w409:string)
                        n190 = Path To String(path=w413) -> (string=w416:string)
                        n191 = Format Into String(format string="Channel: %d\\nps/point: %d\\nns/div: %d\\nAmount of averagings: %d\\n#Sweeps: %d\\nFilter up to (MHz): %f\\nChirp start (MHz): %f\\nAmpl. (dBm): %f\\nf start (MHz): %f\\nf step (MHz): %f\\n#steps: %d\\n", w429, w420, w421, w426, w425, w424, w423, w422, w419, w418, w417) -> (resulting string=w400:string)  [unwired: 2 in, 1 out]
                        n192 = Concatenate Strings(w416, "\\\\" ("string"), w412, "_", "par", ".", w409) -> (w408:string)
                        n193 = case shown="False" w399 {
                          tunnel: [T3."replace or create with confirmation" ("operation (0:open)") T3."replace or create" ("operation (0:open)")] -> w398
                          frame #0 {
                          }
                          frame #1 {
                          }
                        }
                        n194 = String To Path(string=w408) -> (path=w402:path)
                        n195 = Open/Create/Replace File(file path (use dialog)=w402, operation (0:open)=w398, access (0:read/write)=enum16{"read/write", "read-only", "write-only"}."write-only") -> (refnum out=w404:refnum<file>, error out=w407:errorcluster)  [unwired: 3 in, 1 out]
                        n196 = Write to Text File(file (use dialog)=w404, text=w400, error in=w407) -> (refnum out=w405:refnum<file>, error out=w406:errorcluster)  [unwired: 1 in, 1 out]
                        n197 = Close File(refnum=w405, error in=w406) -> (error out=w403:errorcluster)  [unwired: 1 out]
                        n198 = call <vilib>:"Simple Error Handler.vi"("error in (no error)"=w403) -> ()  [unwired: 4 in, 5 out]
                      }
                    }
                    n199 = local write "Stop"(FALSE ("Stop")) -> ()
                  }
                }
              }
            }
          }
        }
        n200 = Wait Until Next ms Multiple(millisecond multiple=u32 150) -> ()  [unwired: 1 out]
      }
    }
    frame #2 {
      n201 = Current VI's Path() -> (path=w441:path)
      n202 = Strip Path(path=w441) -> (stripped path=w442:path)  [unwired: 1 out]
      n203 = Build Path(base path=w442, name or relative path="Data_get.cfg") -> (appended path=w444:path)
      n204 = call "SaveControlValues.vi"("file path"=w444, "vi path"=w441) -> ("error out"=w443:errorcluster)
      n205 = call <vilib>:"Simple Error Handler.vi"("error in (no error)"=w443) -> ()  [unwired: 4 in, 5 out]
    }
  }
